vi "IsReady.vi"(8 "error in (no error)":errorcluster, 11 "reference in":refnum<class "Test_Template.lvclass">) -> (0 "error out":errorcluster, 1 "OK":bool, 3 "reference in":refnum<class "Test_Template.lvclass">)   [LabVIEW 2017]
uses:
  Test_Template.lvclass
  Components/MES_Base.lvlibp/MES_Base.lvclass
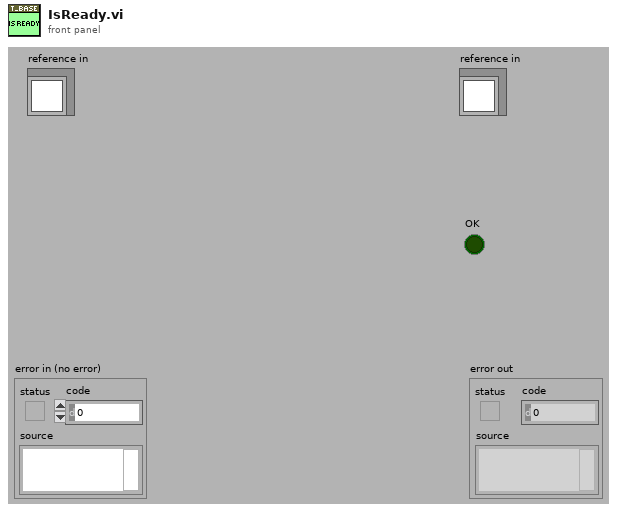
[diagram p1: front panel]
types:
  T1 = typedef "Test_Template.lvlib/Test_Template.lvclass/ObjectAttributes.ctl" = cluster{"Config":T2}
  T2 = typedef "Test_Template.lvlib/Test_Template.lvclass/Config.ctl" = cluster{"default":string}
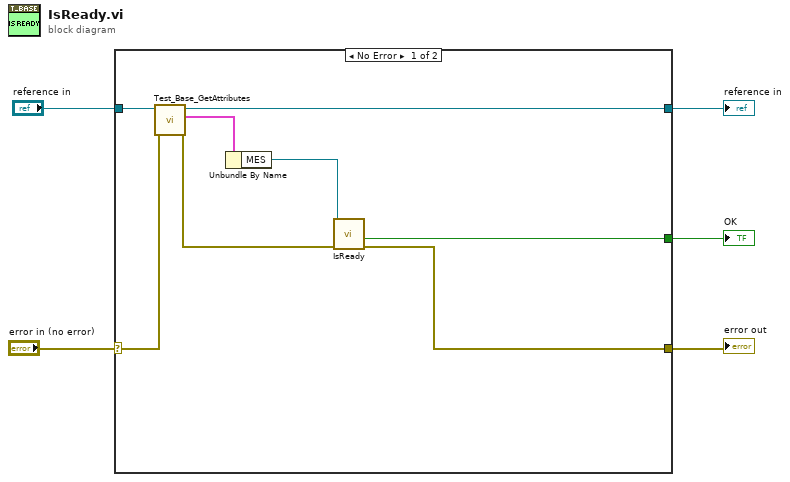
[diagram p0: block diagram]
diagram:
  n1 = case shown="No Error" "error in (no error)" {
    selector: "error in (no error)" -> [w13 w15]
    tunnel: [w7 w15] -> w4
    tunnel: [w10 w14] -> w2
    tunnel: "reference in" -> [w11 w14]
    tunnel: [w6 _] -> w1
    frame No Error {
      n2 = call "Test_Base_GetAttributes.vi"("error in (no error)"=w13, "reference in"=w11) -> ("error out"=w8:errorcluster, "Data"=w12:T1, "reference out"=w10:refnum<class "Test_Template.lvclass">)  [unwired: 6 in, 1 out]
      n3 = Unbundle By Name(w12) -> ("MES"=w9:refnum<class "MES_Base.lvclass">)
      n4 = call-dynamic "IsReady.vi"("error in (no error)"=w8, "reference in"=w9) -> ("error out"=w7:errorcluster, "OK"=w6:bool)  [unwired: 7 in, 1 out]
    }
    frame Error {
    }
  }
  "error out" <- w4
  "reference in" <- w2
  "OK" <- w1
